vi "create new file.vi"(8 "error in":errorcluster, 11 "logging path":path) -> (0 "error out":errorcluster, 3 "tdms file out":refnum<k34>)   [LabVIEW 2013, in "TDMS datalogger runtime.lvclass"]
uses:
  TDMS datalogger runtime.lvclass
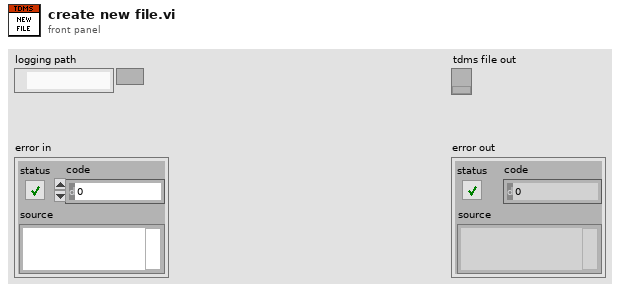
[diagram p1: front panel]
types:
  T1 = enum16{"open", "open or create", "create or replace", "create", "open (read-only)"}
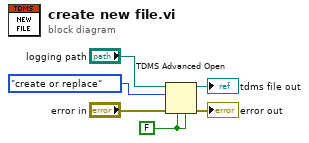
[diagram p0: block diagram]
diagram:
  w5 = FALSE ("disable buffering? (T)")
  n1 = TDMS Advanced Open(4:w5, 6:w5, 8:"error in", 10:T1."create or replace" ("operation (0:open)"), 11:"logging path") -> (0:→"error out":errorcluster, 3:→"tdms file out":refnum<k34>)  [unwired: 1 out]
